vi "Deserialise content.vi"(8 "error in (no error)":errorcluster, 10 "JSON String to decode":string, 11 "object in":refnum<class "execute_reply Message.lvclass">) -> (0 "error out":errorcluster, 3 "object out":refnum<class "execute_reply Message.lvclass">)   [LabVIEW 2018, in "ClientMessaging.lvlib" / "execute_reply Message.lvclass"]
uses:
  execute_reply Message.lvclass
  C:/Users/gavin/Documents/LabVIEW Data/LabVIEW-Bits/Connectivity/Jupyter Client/Base Classes/Reply Message/Reply Message.lvclass
  C:/Users/gavin/Documents/LabVIEW Data/LabVIEW-Bits/Connectivity/Jupyter Client/Base Classes/Message Class/Message Class.lvclass
  execute_reply Message.lvclass/execute_reply Message.ctl
  e0c12bbb-242f-4016-bded-795e34f490a3.vi
  72215ddf-d958-4f96-ab2c-ca2fc19e484f.vi
  60b212bb-439c-44c5-bfa9-ececc24b1901.vi
  e0c12bbb-242f-4016-bded-795e34f490a3.vi/05930108-c59a-4632-a157-4b17e5101890.vi
  e0c12bbb-242f-4016-bded-795e34f490a3.vi/e55128d2-4d16-470f-bb3b-035b1bf60fc4.vi
  e0c12bbb-242f-4016-bded-795e34f490a3.vi/eb8b9d17-24b3-43fb-adf7-da7f7098e852.vi
  <vilib>/JDP Science/JSONtext/Find Item.vi
  72215ddf-d958-4f96-ab2c-ca2fc19e484f.vi/2084b017-59b4-467c-933e-938f004fee73.vi
  72215ddf-d958-4f96-ab2c-ca2fc19e484f.vi/6b5081da-0022-4904-aebe-026c9ad282ae.vi
  60b212bb-439c-44c5-bfa9-ececc24b1901.vi/8b8fb5f0-53a5-4ff1-8143-4d49dfcb960d.vi
  60b212bb-439c-44c5-bfa9-ececc24b1901.vi/c6c4078e-3468-438b-b15d-10f98a904d5f.vi
  60b212bb-439c-44c5-bfa9-ececc24b1901.vi/a3a1a781-fdb8-4566-88f4-a0d13d867993.vi
  <vilib>/JDP Science/JSONtext/String Subset.vi
  <vilib>/JDP Science/JSONtext/Parsing/Parse Full Path or Item Name.vi
  <vilib>/JDP Science/JSONtext/Offset/Find Item Locations by Path.vi
  <vilib>/JDP Science/JSONtext/JSON text to Variant.vi
  Base Classes/Reply Message/Reply Message.lvclass
  Base Classes/Message Class/Message Class.lvclass
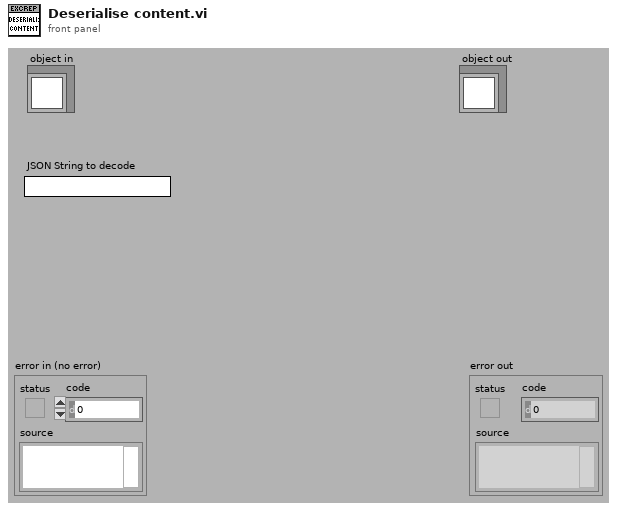
[diagram p1: front panel]
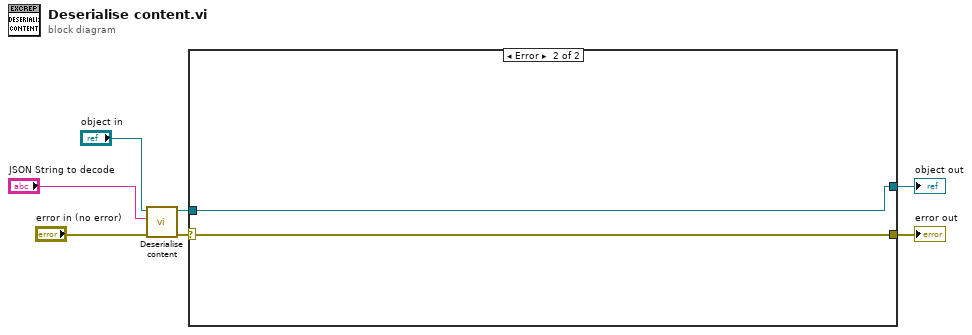
[diagram p0: block diagram]
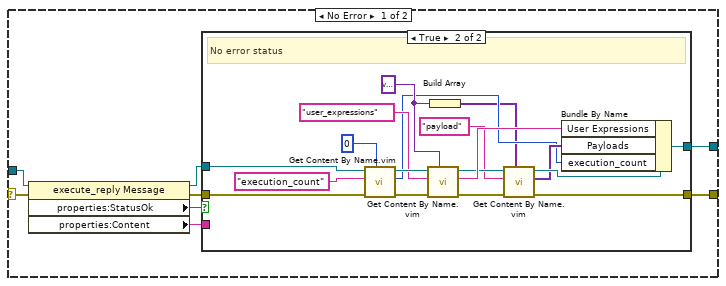
[diagram p2: hidden frame]
diagram:
  n1 = call-parent "Deserialise content.vi"("error in (no error)"="error in (no error)", "JSON String to decode"="JSON String to decode", "object in"="object in") -> ("error out"=w2:errorcluster, "object out"=w1:refnum<class "execute_reply Message.lvclass">)  [unwired: 7 in]
  n2 = case shown="Error" w2 {
    selector: w2 -> [w9 w37]
    tunnel: [w11 w37] -> w7
    tunnel: [w13 w36] -> w5
    tunnel: w1 -> [w8 w36]
    frame No Error {
      n3 = property class="execute_reply Message"(reference=w8, error in=w9) -> (reference out=w12:refnum<class "execute_reply Message.lvclass">, error out=w14:errorcluster, "properties:StatusOk"=w15:bool, "properties:Content"=w10:string)
      n4 = case shown="True" w15 {
        tunnel: w12 -> [w16 w35]
        tunnel: w14 -> [w17 w33]
        tunnel: [w16 w34] -> w13
        tunnel: [w17 w24] -> w11
        tunnel: w10 -> [_ _]
        frame False {
          # "error status handled in parent class"
        }
        frame True {
          w26 = variant ("Type of content")
          # "No error status"
          n5 = call "Get Content By Name.vim"("Type of content"=u32 0, "error in (no error)"=w33, "Name of Content Item"="execution_count" ("Element Name"), "Message In"=w35) -> ("error out"=w30:errorcluster, "Data Out"=w22:u32, "Message Out"=w29:refnum<class "execute_reply Message.lvclass">)  [unwired: 5 in]
          n6 = call "Get Content By Name.vim"("Type of content"=w26, "error in (no error)"=w30, "Name of Content Item"="user_expressions" ("Element Name"), "Message In"=w29) -> ("error out"=w21:errorcluster, "Data Out"=w27:string, "Message Out"=w20:refnum<class "execute_reply Message.lvclass">)  [unwired: 5 in]
          n7 = Build Array(w26) -> (w18:variant[])
          n8 = call "Get Content By Name.vim"("Type of content"=w18, "error in (no error)"=w21, "Name of Content Item"="payload" ("Element Name"), "Message In"=w20) -> ("error out"=w24:errorcluster, "Data Out"=w23:variant[], "Message Out"=w25:refnum<class "execute_reply Message.lvclass">)  [unwired: 5 in]
          n9 = Bundle By Name(cluster=w25, "User Expressions"=w27, "Payloads"=w23, "execution_count"=w22) -> (w34:refnum<class "execute_reply Message.lvclass">)
        }
      }
    }
    frame Error {
    }
  }
  "error out" <- w7
  "object out" <- w5
